vi "Direct Collocation.vi"() -> ()   [LabVIEW 2020]
uses:
  <vilib>/gmath/NumericalOptimization/stopping criteria.ctl
  <vilib>/gmath/NumericalOptimization/cno_bounds.ctl
  <vilib>/gmath/NI_Gmath.lvlib
panel:
  out "error out":errorcluster
  out "XY Graph":cluster{"Time":dbl[], "Control":dbl[]}[](graph)
  in  "stopping criteria":T1={"function tolerance"=1e-06, "parameter tolerance"=1e-06, "max iterations"=100, "max function calls"=1000, "gradient tolerance"=1e-06, "max time (sec)"=-1.0}
  in  "State Bounds":dbl[][](array[numeric])=[[-0.01, 1.01], [-20.0, 20.0]]
  in  "Control Bounds":dbl[][](array[numeric])=[[-50.0, 50.0]]
  in  "Final State Bounds":dbl[][](array[numeric])=[[0.99, 1.01], [-0.01, 0.01]]
  in  "Initial State Bounds":dbl[][](array[numeric])=[[-0.01, 0.01], [-0.01, 0.01]]
  out "minimum":dbl[](array[numeric])
  in  "Final Time Bounds":dbl
  in  "Initial Time Bounds":dbl
  in  "Control":dbl[][](array[numeric])=[[1.0, -1.0]]
  in  "State":dbl[][](array[numeric])=[[0.0, 1.0], [0.0, 0.0]]
  in  "Time":dbl[](array[numeric])=[0.0, 10.0]
  in  "nGrid":dbl=15.0
  # "Initial Guess"
  # "Bounds"
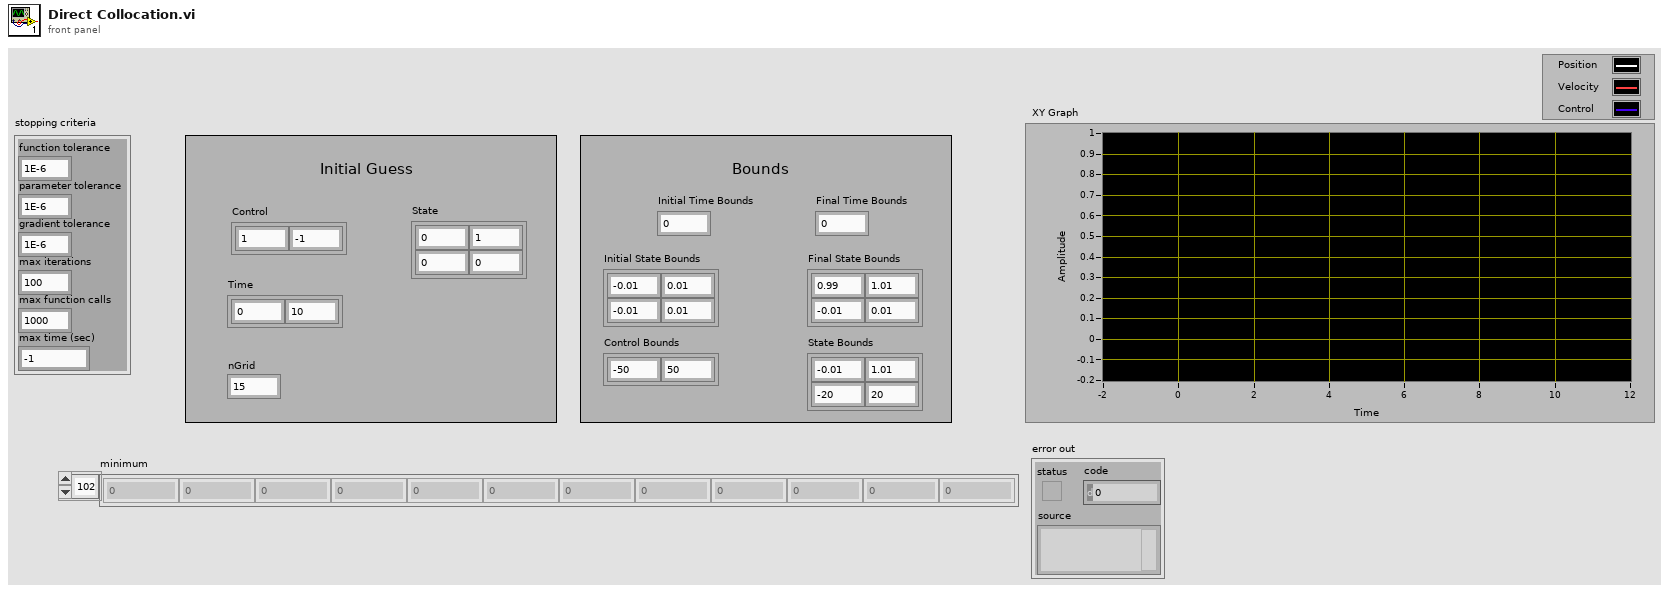
[diagram p1: front panel]
types:
  T1 = typedef "NI_Gmath.lvlib/stopping criteria.ctl" = cluster{"function tolerance":dbl, "parameter tolerance":dbl, "max iterations":i32, "max function calls":i32, "gradient tolerance":dbl, "max time (sec)":dbl}
  T2 = cluster{"nGrid":dbl, "nControl":i32, "nState":i32}
  T3 = typedef "NI_Gmath.lvlib/cno_bounds.ctl" = cluster{"X minimum":dbl[], "X maximum":dbl[], "inequality constraint minimum":dbl[], "inequality constraint maximum":dbl[]}
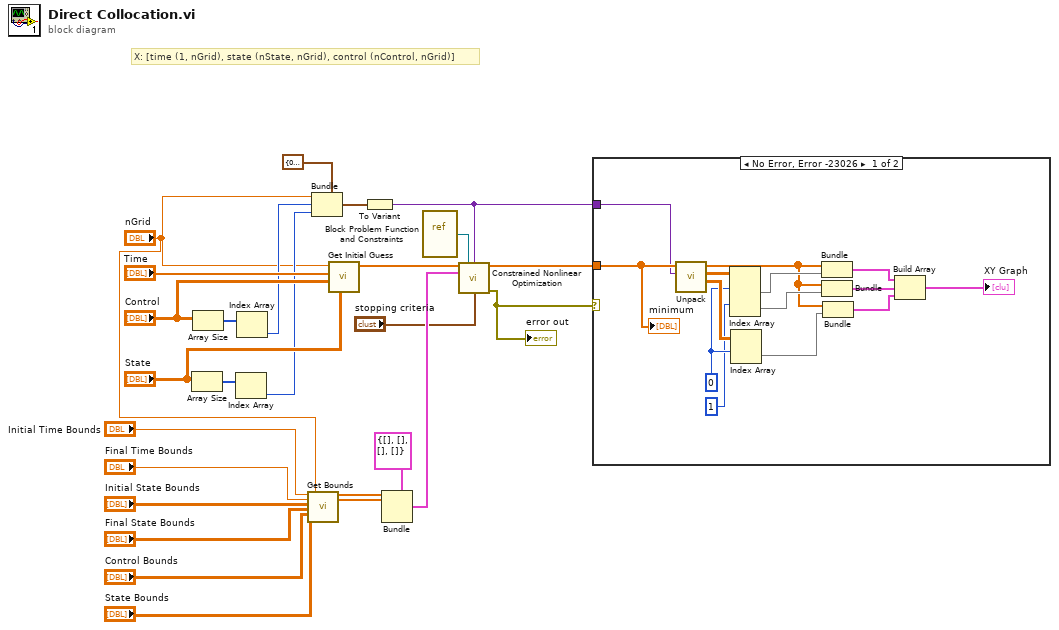
[diagram p0: block diagram]
diagram:
  # "X: [time (1, nGrid), state (nState, nGrid), control (nControl, nGrid)]"
  n1 = Array Size(array="State") -> (size(s)=w26:i32[])
  n2 = Array Size(array="Control") -> (size(s)=w24:i32[])
  n3 = Index Array(array=w26) -> (element=w19:i32)  [unwired: 1 in]
  n4 = Index Array(array=w24) -> (element=w20:i32)  [unwired: 1 in]
  n5 = call "Get Bounds.vi"("Initial Time Bounds"="Initial Time Bounds", "Final Time Bounds"="Final Time Bounds", "Initial State Bounds"="Initial State Bounds", "Final State Bounds"="Final State Bounds", "Control Bounds"="Control Bounds", "State Bounds"="State Bounds", "nGrid"="nGrid") -> ("bLow"=w15:dbl[], "bHigh"=w11:dbl[])  [unwired: 11 in]
  n6 = Bundle(cluster=T2 {"nGrid"=0.0, "nControl"=0, "nState"=0} ("output cluster"), "nGrid"="nGrid", "nControl"=w20, "nState"=w19) -> (w18:T2)
  n7 = call "Get Initial Guess.vi"("State"="State", "Control"="Control", "Time"="Time", "nGrid"="nGrid") -> ("Array"=w21:dbl[])  [unwired: 7 in]
  n8 = To Variant(anything=w18) -> (Variant=w2:variant)
  n9 = Bundle(cluster=T3 {"X minimum"=[], "X maximum"=[], "inequality constraint minimum"=[], "inequality constraint maximum"=[]} ("bounds"), "X minimum"=w15, "X maximum"=w11) -> (w16:T3)  [unwired: 2 in]
  n10 = vi-ref "Block Problem Function and Constraints.vi"() -> (w9:refnum<vi>)
  n11 = call <vilib>:"Constrained Nonlinear Optimization.vi"("start"=w21, "objective and constraint function"=w9, "function data"=w2, "bounds"=w16, "stopping criteria"="stopping criteria") -> ("minimum"=w3:dbl[], "error out"=w1:errorcluster)  [unwired: 6 in, 3 out]
  "error out" <- w1
  n12 = case shown="No Error, Error -23026" w1 {
    tunnel: w3 -> [w40 _]
    tunnel: w2 -> [w39 _]
    frame No Error {
      w36 = 0 ("index (row)")
      n13 = call "Unpack.vi"("data"=w39, "X"=w40) -> ("Control"=w38:dbl[][], "State"=w37:dbl[][], "Time"=w31:dbl[])  [unwired: 7 in]
      n14 = Index Array(array=w37, index (row) #1=w36, index (row) #2=1 ("index (row)")) -> (element #1=w32:dbl[], element #2=w33:dbl[])  [unwired: 2 in]
      n15 = Index Array(array=w38, index (row)=w36) -> (element=w34:dbl[])  [unwired: 1 in]
      n16 = Bundle("Time"=w31, "State"=w32) -> (w30:cluster{"Time":dbl[], "State":dbl[]})  [unwired: 1 in]
      n17 = Bundle("Time"=w31, "State"=w33) -> (w29:cluster{"Time":dbl[], "State":dbl[]})  [unwired: 1 in]
      n18 = Bundle("Time"=w31, "Control"=w34) -> (w28:cluster{"Time":dbl[], "Control":dbl[]})  [unwired: 1 in]
      n19 = Build Array(w30, w29, w28) -> (→"XY Graph":cluster{"Time":dbl[], "Control":dbl[]}[])
      "minimum" <- w40
    }
    frame Default {
    }
  }
